vi "Command Window (GPIB).vi"() -> ()   [LabVIEW 2011]
panel:
  in  "VISA resource name":refnum<visa-resource-name>
  out "CryoCon":bool
  out "Lakeshore":bool
  out "Response":string
  in  "Command":string
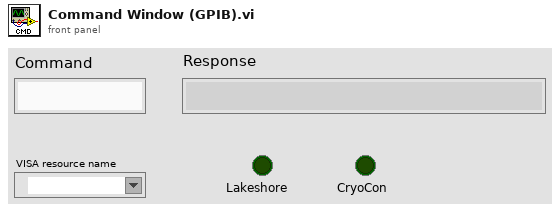
[diagram p1: front panel]
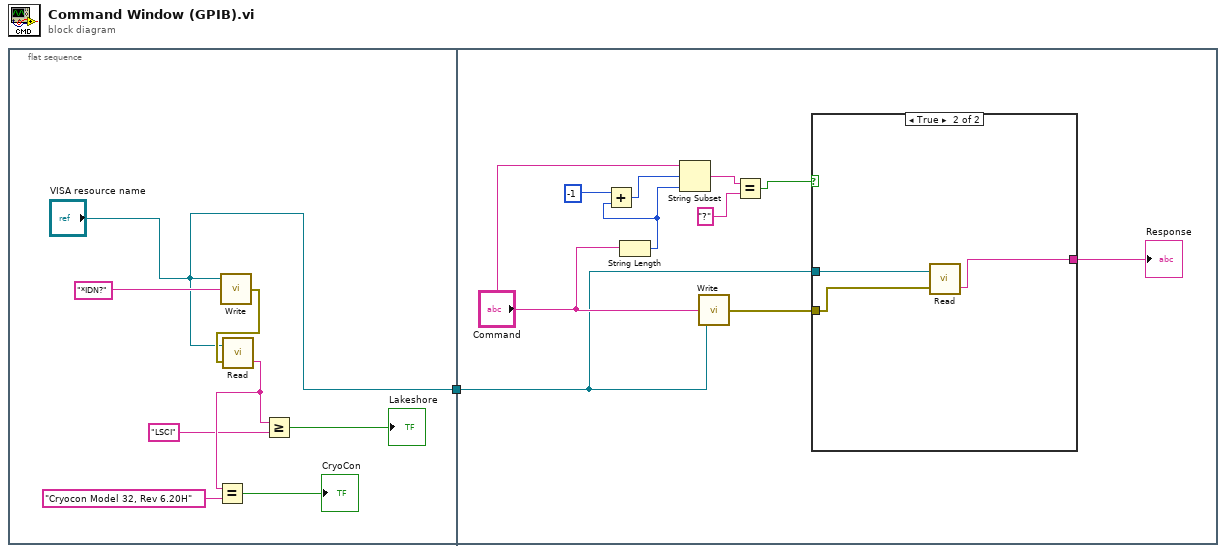
[diagram p0: block diagram]
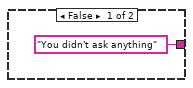
[diagram p2: hidden frame]
diagram:
  n1 = flat-sequence {
    tunnel: ["VISA resource name"] -> w1
    tunnel: w1 -> [w10]
    frame #0 {
      n2 = call "Write.vi"("write buffer"="*IDN?", "VISA resource name"="VISA resource name") -> ("error out"=w7:errorcluster)  [unwired: 1 in]
      n3 = call "Read.vi"("error in (no error)"=w7, "VISA resource name"="VISA resource name") -> ("read buffer"=w5:string)  [unwired: 1 out]
      n4 = Equal?(x=w5, y="Cryocon Model 32, Rev 6.20H") -> (x = y?=→"CryoCon":bool)
      n5 = Greater Or Equal?(x=w5, y="LSCI") -> (x >= y?=→"Lakeshore":bool)
    }
    frame #1 {
      n6 = String Length(string="Command") -> (length=w19:i32)
      n7 = Add(x=-1, y=w19) -> (x+y=w17:i32)
      n8 = String Subset(string="Command", offset (0)=w17, length (rest)=w19) -> (substring=w16:string)
      n9 = call "Write.vi"("write buffer"="Command", "VISA resource name"=w10) -> ("error out"=w12:errorcluster)  [unwired: 1 in]
      n10 = Equal?(x=w16, y="?") -> (x = y?=w14:bool)
      n11 = case shown="True" w14 {
        tunnel: ["You didn't ask anything" ("read buffer") w23] -> w11
        tunnel: w12 -> [_ w22]
        tunnel: w10 -> [_ w21]
        frame False {
        }
        frame True {
          n12 = call "Read.vi"("error in (no error)"=w22, "VISA resource name"=w21) -> ("read buffer"=w23:string)  [unwired: 1 out]
        }
      }
      "Response" <- w11
    }
  }
